vi "Run.vi"(6 "Type y_pred":T1(ring), 7 "Type y_true":T1(ring), 8 "error in (no error)":errorcluster caption="entrée d'erreur (pas d'erreur)", 9 "y_pred":string[][](array[string]), 10 "y_true":string[][](array[string]), 11 "Zero_One_Loss.lvclass":refnum<class "Zero_One_Loss.lvclass">) -> (0 "error out":errorcluster caption="sortie d'erreur", 2 "String Data":string, 3 "Zero_One_Loss.lvclass":refnum<class "Zero_One_Loss.lvclass">)   [LabVIEW 2020, in "Zero_One_Loss.lvclass"]
doc: "Returns : \n\n- loss : float or int,\nIf normalize == True, return the fraction of misclassifications (float), else it returns the number of misclassifications (int)"
uses:
  Zero_One_Loss.lvclass
  Zero_One_Loss.lvclass/Zero_One_Loss.ctl
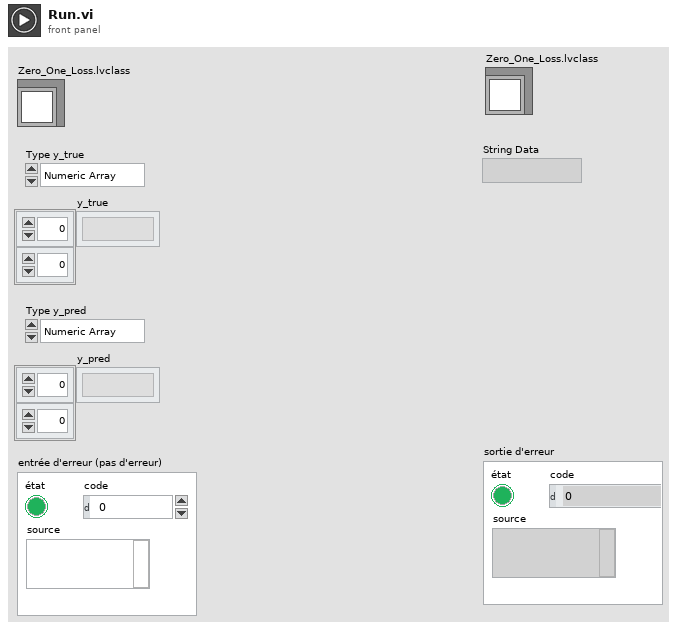
[diagram p1: front panel]
types:
  T1 = enum16{"Numeric Array", "String Array", "Sparse"}
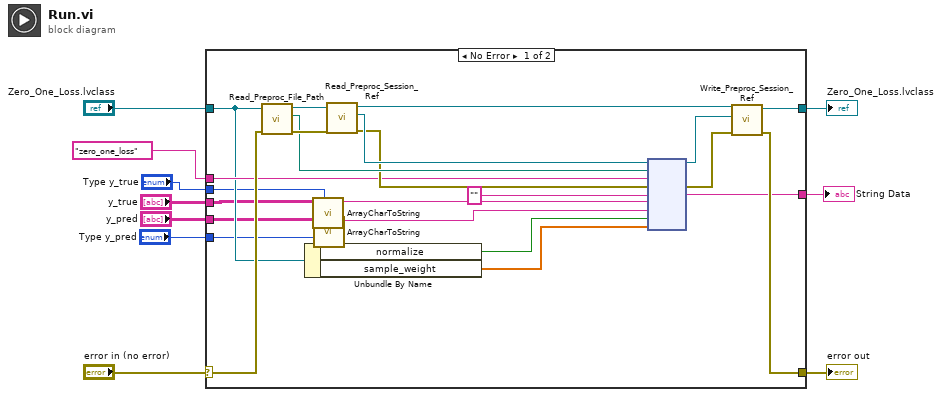
[diagram p0: block diagram]
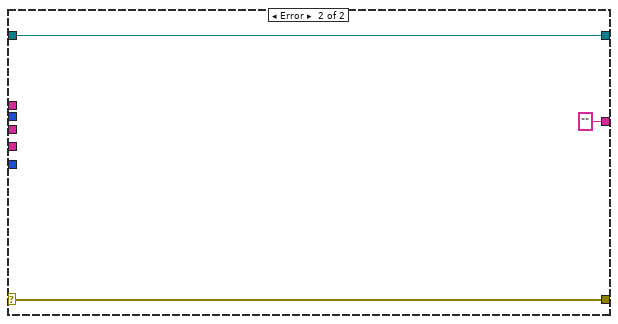
[diagram p2: hidden frame]
diagram:
  n1 = case shown="No Error" "error in (no error)" {
    selector: "error in (no error)" -> [w22 w36]
    tunnel: [w23 w36] -> w9
    tunnel: [w24 w35] -> w7
    tunnel: "Zero_One_Loss.lvclass" -> [w19 w35]
    tunnel: "zero_one_loss" -> [w21 _]
    tunnel: [w20 ""] -> w6
    tunnel: "y_true" -> [w16 _]
    tunnel: "y_pred" -> [w15 _]
    tunnel: "Type y_true" -> [w12 _]
    tunnel: "Type y_pred" -> [w11 _]
    frame No Error {
      n2 = call-dynamic "Read_Preproc_File_Path.vi"("error in (no error)"=w22, "Python in"=w19) -> ("error out"=w32:errorcluster, "File_Path"=w31:path, "Python out"=w33:refnum<class "Zero_One_Loss.lvclass">)  [unwired: 7 in]
      n3 = Unbundle By Name(w19) -> ("normalize"=w18:bool, "sample_weight"=w17:dbl[])
      n4 = call "ArrayCharToString.vi"("Type"=w12, "TAB"=w16) -> ("Instruction"=w14:string)  [unwired: 9 in]
      n5 = call "ArrayCharToString.vi"("Type"=w11, "TAB"=w15) -> ("Instruction"=w13:string)  [unwired: 9 in]
      n6 = call-dynamic "Read_Preproc_Session_Ref.vi"("error in (no error)"=w32, "Python in"=w33) -> ("error out"=w29:errorcluster, "Session_ref"=w30:refnum<k35>, "Python out"=w28:refnum<class "Zero_One_Loss.lvclass">)  [unwired: 7 in]
      n7 = node(w30, w31, w21, w29, "", w14, w13, w18, w17) -> (w26:refnum<k35>, w27:errorcluster, w20:string)  [unwired: 4 in, 2 out]
      n8 = call-dynamic "Write_Preproc_Session_Ref.vi"("error in (no error)"=w27, "Session_ref"=w26, "Python in"=w28) -> ("error out"=w23:errorcluster, "Python out"=w24:refnum<class "Zero_One_Loss.lvclass">)  [unwired: 7 in]
    }
    frame Error {
    }
  }
  "error out" <- w9
  "Zero_One_Loss.lvclass" <- w7
  "String Data" <- w6
